vi "Periodic Tasks.vi"(8 "error in":errorcluster) -> ()   [LabVIEW 2016]
doc: "This VI runs in parallel to other tasks. It can contain as many user-defined periodic loops as you need. These can carry out PID or other sorts of timed response."
uses:
  <vilib>/Rock Robotics/WPI/Utilities/WPI_GetSetVariantRefNum.vi
  <vilib>/Rock Robotics/Network Tables/NT Write Number.vi
  <vilib>/Rock Robotics/WPI/Ultrasonic/WPI_SonarMB1010AnalogRefNum Registry Get.vi
  <vilib>/Rock Robotics/WPI/Ultrasonic/WPI_SonarMB1010AnalogGetRange.vi
  <vilib>/Rock Robotics/WPI/ThirdParty/Sensors/ADIS16448 IMU/ADIS16448_IMU.lvlib
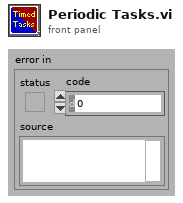
[diagram p1: front panel]
types:
  T1 = typedef "WPI_JoystickDevRef.ctl" = cluster{"Device":T2}
  T2 = typedef "WPI_JoystickDeviceEnum.ctl" = enum16{"USB 0", "USB 1", "USB 2", "USB 3", "USB 4", "USB 5"}
  T3 = typedef "WPI_RobotDriveDevRef.ctl" = cluster{"DevStatus":errorcluster, "Motors[]":T4[], "Square Inputs":bool, "Max Output":dbl}
  T4 = typedef "WPI_MotorControlDeviceRef.ctl" = cluster{"DeviceStatus":errorcluster, "Type":T5, "PWM":cluster{"PWM Channel":T6, "DeadBand":T7}, "CAN":cluster{"Device Number":u8, "SetOutput VI Ref":variant, "GetOutput VI Ref":variant, "Enable VI Ref":variant, "Disable VI Ref":variant, "Data":variant}, "Invert":bool}
  T5 = typedef "WPI_MotorControlType.ctl" = enum16{"PWM", "CAN"}
  T6 = typedef "FPGA_DIOPWMChannel.ctl" = enum8{"PWM 0", "PWM 1", "PWM 2", "PWM 3", "PWM 4", "PWM 5", "PWM 6", "PWM 7", "PWM 8", "PWM 9", "PWM MXP 0", "PWM MXP 1", "PWM MXP 2", "PWM MXP 3", "PWM MXP 4", "PWM MXP 5", "PWM MXP 6", "PWM MXP 7", "PWM MXP 8", "PWM MXP 9", "Invalid"}
  T7 = typedef "WPI_PWMDeadband.ctl" = cluster{"Name":string, "maxPositivePwm":i32, "minPositivePwm":i32, "centerPwm":i32, "maxNegativePwm":i32, "minNegativePwm":i32, "angularRange":u16}
  T8 = typedef "WPI_SonarMB1010AnalogDeviceRef.ctl" = cluster{"AIDeviceRef":T9, "Scaling factor (V/in)":dbl, "Average Bits":u8}
  T9 = typedef "WPI_AnalogChannelDevRef.ctl" = cluster{"DevStatus":errorcluster, "Analog Channel":T10}
  T10 = typedef "FPGA_AIChannel.ctl" = enum8{"AI 0", "AI 1", "AI 2", "AI 3", "AI MXP 0", "AI MXP 1", "AI MXP 2", "AI MXP 3", "Invalid"}
  T11 = typedef "ADIS16448_IMU.lvlib/ADI_IMU_ADIS16448_InterruptDevRef.ctl" = cluster{"ADI IMU DevRef":T12, "InterruptRef":T14}
  T12 = typedef "ADIS16448_IMU.lvlib/ADI_IMU_ADIS16448_IMUDevRef.ctl" = cluster{"DevStatus":errorcluster, "Handle":i32, "SPI Bus":T13, "Device Found":bool, "Device Ready":bool, "Yaw Axis":enum16{"X", "Y", "Z"}, "AHRS Algorithm":enum16{"Complementary", "Madgwick"}, "Serial":u16, "Lot ID 2":u16, "Lot ID 1":u16, "Product ID":u16}
  T13 = typedef "spi_bus.ctl" = enum16{"SPI On-Board, CS0", "SPI On-Board, CS1", "SPI On-Board, CS2", "SPI On-Board, CS3", "SPI MXP", "Invalid"}
  T14 = typedef "WPI_InterruptRef.ctl" = cluster{"DevStatus":errorcluster, "InterruptIndex":T15}
  T15 = typedef "FPGA_InterruptIndex.ctl" = enum8{"0", "1", "2", "3", "4", "5", "6", "7", "Invalid"}
  T16 = cluster{"JoystickDevRef":T1, "RobotDriveDevRef":T3}
  T17 = cluster{"X Angle":dbl, "Y Angle":dbl, "Z Angle":dbl}
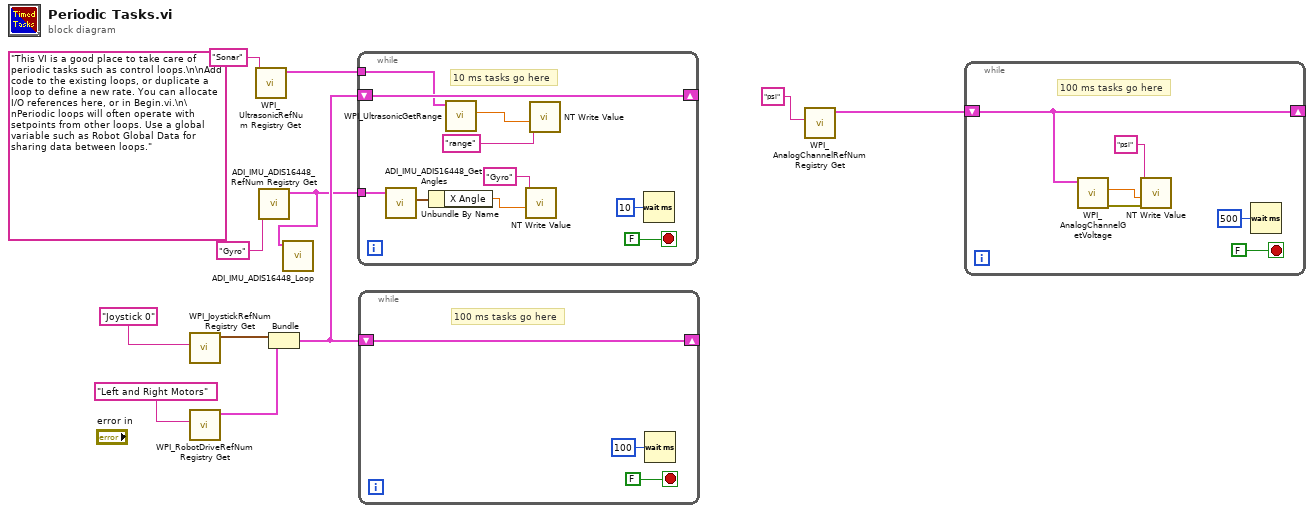
[diagram p0: block diagram]
diagram:
  (unwired) "This VI is a good place to take care of periodic tasks such as control loops.\n\nAdd code to the existing loops, or duplicate a loop to define a new rate. You can allocate I/O references here, or in Begin.vi.\n\nPeriodic loops will often operate with setpoints from other loops. Use a global variable such as Robot Global Data for sharing data between loops."
  n1 = call <vilib>:"WPI_JoystickRefNum Registry Get.vi"("refnum name"="Joystick 0") -> ("JoystickDevRef"=w9:T1)  [unwired: 1 in, 9 out]
  n2 = call <vilib>:"WPI_RobotDriveRefNum Registry Get.vi"("refnum name"="Left and Right Motors") -> ("RobotDriveDevRef"=w8:T3)  [unwired: 1 in, 9 out]
  n3 = call-poly <vilib>:"WPI_UltrasonicRefNum Registry Get.vi"("refnum name"="Sonar") -> ("SonarMB1010AnalogDevRef"=w4:T8)  [unwired: 9 in, 1 out]
  n4 = call <vilib>:"ADI_IMU_ADIS16448_RefNum Registry Get.vi"("refnum name"="Gyro") -> ("ADI IMU Interrupt DevRef"=w1:T11)  [unwired: 9 in, 1 out]
  n5 = Bundle("JoystickDevRef"=w9, "RobotDriveDevRef"=w8) -> (w5:T16)  [unwired: 1 out]
  n6 = call <vilib>:"ADI_IMU_ADIS16448_Loop.vi"("ADI_IMU_DevRef"=w1) -> ()  [unwired: 9 in, 2 out]
  n7 = while {
    shift-right: [w19] -> _
    shift-left: w5 -> [w19]
    tunnel: w4 -> [w18]
    tunnel: w1 -> [w15]
    stop <- FALSE stop-if-true
    # "10 ms tasks go here"
    n8 = call <vilib>:"ADI_IMU_ADIS16448_Get Angles.vi"("ADI IMU Interrupt DevRef"=w15) -> ("IMU Angles Out"=w14:T17)  [unwired: 7 in, 3 out]
    n9 = Unbundle By Name(w14) -> ("X Angle"=w13:dbl)
    n10 = call-poly <vilib>:"WPI_UltrasonicGetRange.vi"("SonarMB1010AnalogDevRef"=w18) -> ("Distance"=w17:dbl)  [unwired: 8 in, 2 out]
    n11 = call-poly <vilib>:"NT Write Value.vi"("Numeric"=w13, "Name"="Gyro") -> ()  [unwired: 9 in, 1 out]
    n12 = call-poly <vilib>:"NT Write Value.vi"("Numeric"=w17, "Name"="range") -> ()  [unwired: 9 in, 1 out]
    n13 = Wait (ms)(milliseconds to wait=u32 10) -> ()  [unwired: 1 out]
  }
  n14 = while {
    shift-right: [w22] -> _
    shift-left: w5 -> [w22]
    stop <- FALSE stop-if-true
    # "100 ms tasks go here"
    n15 = Wait (ms)(milliseconds to wait=u32 100) -> ()  [unwired: 1 out]
  }
  n16 = call <vilib>:"WPI_AnalogChannelRefNum Registry Get.vi"("refnum name"="psi") -> ("AIDeviceRef"=w7:T9)  [unwired: 9 in, 1 out]
  n17 = while {
    shift-right: [w28] -> _
    shift-left: w7 -> [w28]
    stop <- FALSE stop-if-true
    # "100 ms tasks go here"
    n18 = call <vilib>:"WPI_AnalogChannelGetVoltage.vi"("AIDeviceRef"=w28) -> ("error out"=w27:errorcluster, "Voltage"=w26:dbl)  [unwired: 8 in, 1 out]
    n19 = call-poly <vilib>:"NT Write Value.vi"("error in"=w27, "Numeric"=w26, "Name"="psi") -> ()  [unwired: 8 in, 1 out]
    n20 = Wait (ms)(milliseconds to wait=u32 500) -> ()  [unwired: 1 out]
  }
